vi "checkInputStringIsNotEmpty.vi"(8 "error in (no error)":errorcluster, 10 "inputString":string, 11 "TcpServerBase in":refnum<class "TcpServerBase.lvclass">) -> (0 "error out":errorcluster, 3 "TcpServerBase out":refnum<class "TcpServerBase.lvclass">)   [LabVIEW 2018, in "TcpServerBase.lvclass"]
doc: "Check the input string: If is not empty, the input is an unknown message and is sent as a GenRead user event to the user. If is empty, nothing is done in this VI, and the GenRead user event is used to let the user know about the connection status of TCP clients."
uses:
  TcpServerBase.lvclass
  typedef/connStatusCluster.ctl
  TcpServerBase.lvclass/TcpServerBase.ctl
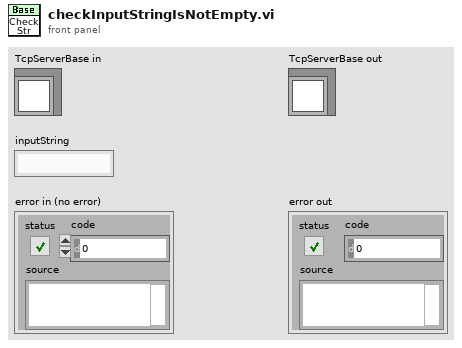
[diagram p1: front panel]
types:
  T1 = typedef "TcpServerBase.lvclass/connStatusCluster.ctl" = cluster{"connStatus":bool, "message":string}
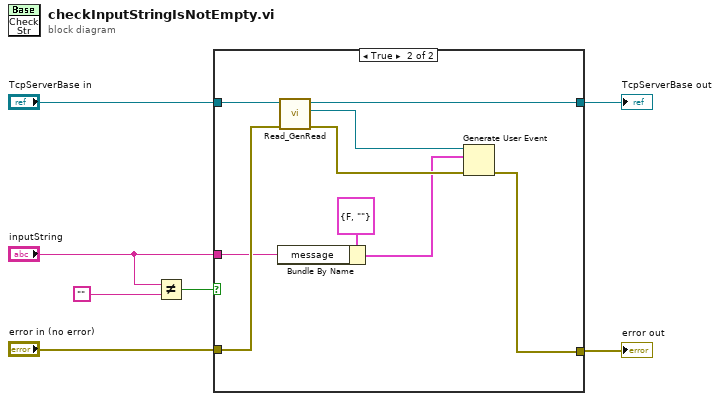
[diagram p0: block diagram]
diagram:
  n1 = Not Equal?(x="inputString", y="") -> (x != y?=w3:bool)
  n2 = case shown="True" w3 {
    tunnel: "error in (no error)" -> [w9 w16]
    tunnel: [w8 w15] -> w6
    tunnel: "TcpServerBase in" -> [w8 w14]
    tunnel: [w9 w13] -> w4
    tunnel: "inputString" -> [_ w10]
    frame False {
    }
    frame True {
      n3 = Bundle By Name(cluster=T1 {"connStatus"=FALSE, "message"=""} ("event data"), "message"=w10) -> (w12:T1)
      n4 = call "Read_GenRead.vi"("error in (no error)"=w16, "TcpServerBase in"=w14) -> ("error out"=w17:errorcluster, "GenRead"=w18:refnum<user-event>, "TcpServerBase out"=w15:refnum<class "TcpServerBase.lvclass">)  [unwired: 7 in]
      n5 = Generate User Event(user event=w18, event data cluster=w12, error in=w17) -> (error out=w13:errorcluster)  [unwired: 1 in, 1 out]
    }
  }
  "TcpServerBase out" <- w6
  "error out" <- w4
